vi "Export File - Common Block XML.vi"(4 "Common":T1, 6 "RootNode in":refnum<k24>, 7 "XmlDocument in":refnum<k24>, 8 "error in (no error)":errorcluster) -> (0 "error out":errorcluster)   [LabVIEW 2016, in "UDP-Custom-Device System Explorer.lvlib"]
uses:
  UDP-Custom-Device System Explorer.lvlib
  <vilib>/NI Veristand/Custom Device API/Custom Device Item Info.ctl
  System.Xml
  <vilib>/NI VeriStand/Custom Device API/Custom Device API.lvlib
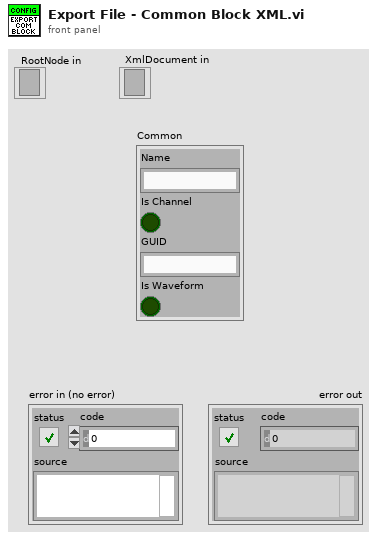
[diagram p1: front panel]
types:
  T1 = typedef "Custom Device API.lvlib/Custom Device Item Info.ctl" = cluster{"Name":string, "Is Channel":bool, "GUID":string, "Is Waveform":bool}
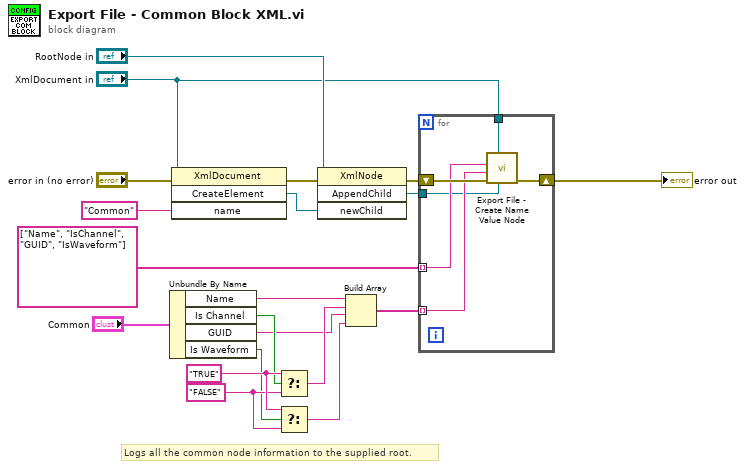
[diagram p0: block diagram]
diagram:
  w8 = "FALSE" ("name")
  w9 = "TRUE" ("name")
  # "Logs all the common node information to the supplied root."
  n1 = Unbundle By Name("Common") -> ("Name"=w10:string, "Is Channel"=w7:bool, "GUID"=w4:string, "Is Waveform"=w6:bool)
  n2 = invoke class="XmlDocument" method="CreateElement"(reference="XmlDocument in", error in="error in (no error)", "name"="Common") -> (error out=w16:errorcluster, "CreateElement"=w15:refnum<k24>)  [unwired: 1 in, 2 out]
  n3 = Select(t=w9, s=w7, f=w8) -> (s? t:f=w5:string)
  n4 = Select(t=w9, s=w6, f=w8) -> (s? t:f=w3:string)
  n5 = invoke class="XmlNode" method="AppendChild"(reference="RootNode in", error in=w16, "newChild"=w15) -> (error out=w14:errorcluster, "AppendChild"=w13:refnum<k24>)  [unwired: 1 in, 2 out]
  n6 = Build Array(w10, w5, w4, w3) -> (w2:string[])
  n7 = for {
    tunnel: string[] ["Name", "IsChannel", "GUID", "IsWaveform"] ("name") -> [w24] mode=indexing
    tunnel: w2 -> [w23] mode=indexing
    shift-right: [w22] -> w12
    shift-left: w14 -> [w26]
    tunnel: "XmlDocument in" -> [w25]
    tunnel: w13 -> [w21]
    n8 = call "Export File - Create Name Value Node.vi"("RootNode in"=w21, "XmlDocument in"=w25, "error in (no error)"=w26, "Value"=w23, "Name"=w24) -> ("error out"=w22:errorcluster)  [unwired: 6 in]
  }
  "error out" <- w12
